vi "PassOrFail (SubVI).vi"(7 "index (row)":i32, 8 "error in (no error)":errorcluster, 9 "Data in":dbl format="%#_13g", 10 "Pass?Fail":bool, 11 "Table in":refnum<vi>) -> (0 "error out":errorcluster)   [LabVIEW 2017]
uses:
  <vilib>/Utility/miscctls.llb/LVRowAndColumnTypeDef.ctl
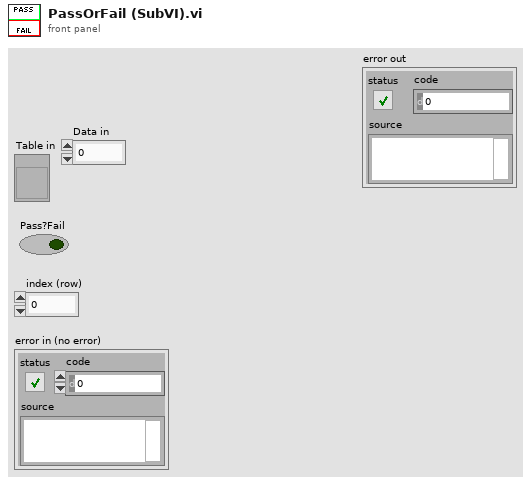
[diagram p1: front panel]
types:
  T1 = typedef "LVRowAndColumnTypeDef.ctl" = cluster{"Row":i32, "Column":i32}
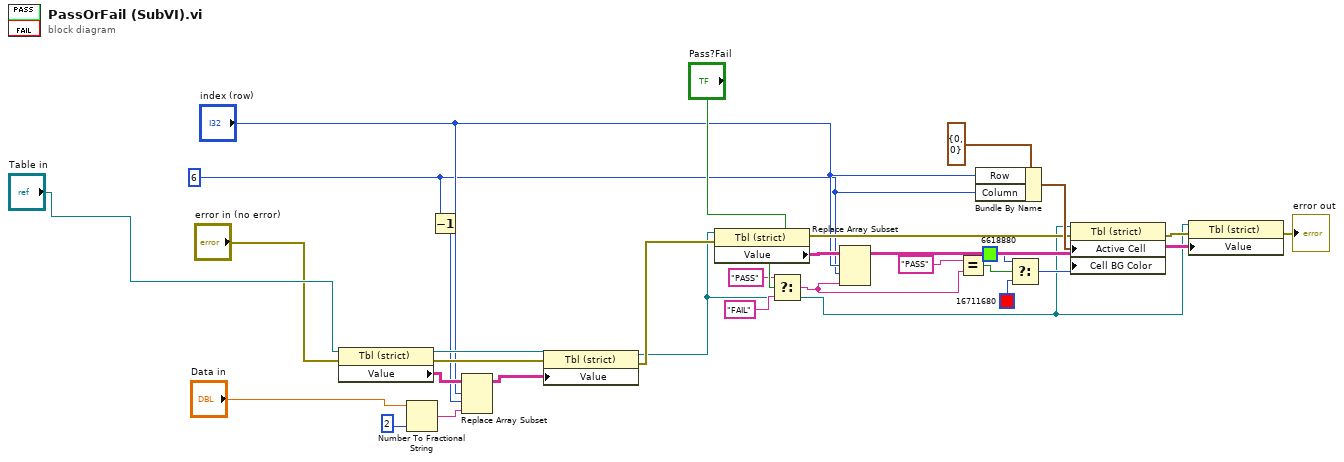
[diagram p0: block diagram]
diagram:
  w4 = 6 ("disabled index (col)")
  n1 = property class="Tbl (strict)"(reference="Table in", error in="error in (no error)") -> (reference out=w8:refnum<vi>, error out=w10:errorcluster, "Value"=w14:string[][])
  n2 = Number To Fractional String(number="Data in", precision (6)=i16 2) -> (F-format string=w6:string)  [unwired: 2 in]
  n3 = Decrement(x=w4) -> (x-1=w3:i32)
  n4 = Replace Array Subset(array=w14, new element=w6, index (row)="index (row)", index (col)=w3) -> (w13:string[][])
  n5 = property class="Tbl (strict)"(reference=w8, error in=w10, "Value"=w13) -> (reference out=w7:refnum<vi>, error out=w9:errorcluster)
  n6 = property class="Tbl (strict)"(reference=w7, error in=w9) -> (error out=w24:errorcluster, "Value"=w21:string[][])  [unwired: 1 out]
  n7 = Select(t="PASS" ("x"), s="Pass?Fail", f="FAIL" ("x")) -> (s? t:f=w27:string)
  n8 = Replace Array Subset(array=w21, new element=w27, index (row)="index (row)", index (col)=w4) -> (w22:string[][])
  n9 = Equal?(x="PASS", y=w27) -> (x = y?=w16:bool)
  n10 = Bundle By Name(cluster=T1 {"Row"=0, "Column"=0} ("Active Cell:Active Cell"), "Row"="index (row)", "Column"=w4) -> (w30:T1)
  n11 = Select(t=u32 6618880, s=w16, f=u32 16711680) -> (s? t:f=w20:u32)
  n12 = property class="Tbl (strict)"(reference=w7, error in=w24, "Active Cell"=w30, "Cell BG Color"=w20) -> (error out=w23:errorcluster)  [unwired: 1 out]
  n13 = property class="Tbl (strict)"(reference=w7, error in=w23, "Value"=w22) -> (error out=→"error out":errorcluster)  [unwired: 1 out]
